vi "NM GlobalTest.vi"() -> ()   [LabVIEW 2010] (continued)
            tunnel: [_ w3958] -> w3939
            tunnel: [_ w3957] -> w3938
            tunnel: [_ w3956] -> w3937
            tunnel: w3936 -> [w3946 _]
            tunnel: [FALSE _] -> w3935
            frame #0 {
              n819 = for {
                N: 5 -> [_]
                tunnel: w3946 -> [w3954]
                n820 = Wait Until Next ms Multiple(millisecond multiple=w3954) -> ()  [unwired: 1 out]
                "Props" <- TRUE
              }
              n821 = case shown="\"DAQmx\"" w3944 {
                frame "ULx", Default {
                }
                frame "DAQmx" {
                  n822 = local write "Burst"("Burst 2") -> ()
                  n823 = local write "Edge"("Edge 2") -> ()
                  n824 = local write "Type"("Type 2") -> ()
                  n825 = local write "SIO"("SIO 2") -> ()
                  n826 = local write "DoWord"("DoWord 2") -> ()
                  n827 = local write "DiWord"("Word 2") -> ()
                }
              }
            }
            frame #1 {
              n828 = case shown="\"Get Properties\", Default" "GetSet" {
                tunnel: w3960 -> [w3970 w5157]
                tunnel: w3962 -> [w3969 w5161]
                tunnel: w3959 -> [w3968 w5160]
                tunnel: w3961 -> [w3967 w5156]
                tunnel: [w3966 w5154] -> w3958
                tunnel: [w3964 w5158] -> w3956
                tunnel: [w3965 w5159] -> w3957
                frame "Get Properties", Default {
                  n829 = stacked-sequence {
                    seq-local: [w3976 _] -> [_ w4127]
                    seq-local: [w3975 _] -> [_ w4126]
                    seq-local: [w3974 _] -> [_ w4125]
                    tunnel: w3970 -> [w3978 _]
                    tunnel: w3969 -> [w3973 w4129]
                    tunnel: w3968 -> [w3972 _]
                    tunnel: w3967 -> [w3977 _]
                    tunnel: [_ w4128] -> w3966
                    tunnel: [_ w4124] -> w3965
                    tunnel: [_ w4123] -> w3964
                    frame #0 {
                      n830 = for {
                        N: 3 -> [_]
                        tunnel: w3973 -> [w3989]
                        shift-right: [w3983] -> w3976
                        shift-left: w3972 -> [w3980]
                        shift-right: [w3984] -> w3975
                        shift-left: w3978 -> [w3981]
                        shift-right: [w3985] -> w3974
                        shift-left: w3977 -> [w3994]
                        i -> [w3993]
                        n831 = case shown="2" w3993 {
                          tunnel: [w4019 w4023 w4027] -> w3992
                          frame 0, Default {
                            n832 = Select(t=1, s="Chans", f=0) -> (s? t:f=w4019:i32)
                          }
                          frame 1 {
                            n833 = Select(t=2, s="Done 2", f=0) -> (s? t:f=w4023:i32)
                          }
                          frame 2 {
                            n834 = Select(t=3, s="Err", f=0) -> (s? t:f=w4027:i32)
                          }
                        }
                        n835 = Not A Number/Path/Refnum?(number/path/refnum=w3981) -> (NaN/Path/Refnum?=w3979:bool)
                        n836 = Not A Number/Path/Refnum?(number/path/refnum=w3980) -> ()  [unwired: 1 out]
                        n837 = case shown="2" w3992 {
                          tunnel: w3981 -> [w4032 w4042 w4081 w4100]
                          tunnel: w3994 -> [w4031 w4038 w4080 w4102]
                          tunnel: [w4033 w4041 w4079 w4099] -> w3988
                          tunnel: [w4032 w4040 w4078 w4096] -> w3987
                          tunnel: [w4031 w4044 w4077 w4095] -> w3986
                          tunnel: w3989 -> [_ w4039 w4076 w4098]
                          tunnel: w3980 -> [w4033 w4043 w4075 w4101]
                          tunnel: [_ w4037 _ _] -> w3990
                          tunnel: w3979 -> [_ w4035 _ w4094]
                          frame 0, Default {
                          }
                          frame 1 {
                            n838 = case shown="\"ULx\", Default" w4039 {
                              tunnel: w4042 -> [w4053 w4073]
                              tunnel: [w4052 w4068] -> w4036
                              tunnel: [w4051 w4071] -> w4044
                              tunnel: [w4050 w4073] -> w4040
                              tunnel: [w4049 w4069] -> w4041
                              tunnel: w4043 -> [w4049 w4070]
                              tunnel: w4038 -> [w4048 w4072]
                              tunnel: [w4047 w4067] -> w4037
                              tunnel: w4035 -> [w4046 _]
                              tunnel: [w4045 w4066] -> w4034
                              frame "ULx", Default {
                                n839 = case shown="False" w4046 {
                                tunnel: w4053 -> [w4054 w4063]
                                tunnel: [w4056 u32 0 ("NumberOfChannels")] -> w4052
                                tunnel: [w4057 w4064] -> w4051
                                tunnel: [w4058 w4063] -> w4050
                                tunnel: w4048 -> [w4060 w4064]
                                tunnel: [w4059 TRUE ("Done")] -> w4047
                                tunnel: [w4055 ""] -> w4045
                                frame False {
                                n840 = call "TaskProps.vi"("task in"=w4054, "error in (no error)"=w4060) -> ("task out"=w4058:refnum<k24>, "NumberOfChannels"=w4056:u32, "Done"=w4059:bool, "error out"=w4057:errorcluster, "DeviceName"=w4055:string)  [unwired: 1 in]
                                }
                                frame True {
                                }
                                }
                              }
                              frame "DAQmx" {
                                n841 = property class="DAQmx Task"(reference=w4070, error in=w4072) -> (reference out=w4069:refnum<k21>, error out=w4071:errorcluster, "NumChans"=w4068:u32, "Done"=w4067:bool, "Name"=w4066:refnum<k21>)
                              }
                            }
                            "Done" <- w4037
                            "NumChans" <- w4036
                            "DevName" <- w4034
                          }
                          frame 2 {
                            n842 = case shown="\"ULx\", Default" w4076 {
                              tunnel: w4081 -> [w4082 w4093]
                              tunnel: [w4085 w4091] -> w4077
                              tunnel: [w4086 w4093] -> w4078
                              tunnel: [w4087 w4092] -> w4079
                              tunnel: w4075 -> [w4087 w4089]
                              tunnel: w4080 -> [w4083 w4088]
                              tunnel: [w4084 w4090] -> w4074
                              frame "ULx", Default {
                                n843 = call <vilib>:"ULx Is Task Done.vi"("task in"=w4082, "error in"=w4083) -> ("task out"=w4086:refnum<k24>, "task done?"=w4084:bool, "error out"=w4085:errorcluster)  [unwired: 11 in]
                              }
                              frame "DAQmx" {
                                n844 = call <vilib>:"DAQmx Is Task Done.vi"("task/channels in"=w4089, "error in"=w4088) -> ("task out"=w4092:refnum<k21>, "task done?"=w4090:bool, "error out"=w4091:errorcluster)  [unwired: 11 in]
                              }
                            }
                            "IT Done" <- w4074
                          }
                          frame 3 {
                            n845 = case shown="\"ULx\", Default" w4098 {
                              tunnel: w4100 -> [w4110 w4122]
                              tunnel: [w4105 w4120] -> w4095
                              tunnel: [w4104 w4122] -> w4096
                              tunnel: [w4109 w4121] -> w4099
                              tunnel: w4101 -> [w4109 w4121]
                              tunnel: w4102 -> [w4108 w4120]
                              tunnel: [w4107 w4119] -> w4097
                              tunnel: w4094 -> [w4103 _]
                              frame "ULx", Default {
                                n846 = case shown="False" w4103 {
                                tunnel: w4110 -> [w4115 w4118]
                                tunnel: w4108 -> [w4114 w4117]
                                tunnel: [w4113 0 ("ErrorCode")] -> w4107
                                tunnel: [w4112 w4117] -> w4106
                                tunnel: [w4111 w4118] -> w4104
                                frame False {
                                n847 = property class="IOTask"(reference=w4115, error in=w4114) -> (reference out=w4111:refnum<k24>, error out=w4112:errorcluster, "ErrorCode"=w4113:i32)
                                }
                                frame True {
                                }
                                }
                                n848 = call <vilib>:"ULx Get Error Info.vi"("error in"=w4106, "ErrorCode"=w4107, "task in"=w4104) -> ("error out"=w4105:errorcluster)  [unwired: 8 in]
                              }
                              frame "DAQmx" {
                                n849 = Unbundle By Name(w4120) -> ("code"=w4119:i32)
                              }
                            }
                            "ErrorCode" <- w4097
                          }
                        }
                        n850 = And(x=w3990, y="Restart\nWhen\nDone") -> (x .and. y?=w3991:bool)
                        n851 = case shown="True" w3991 {
                          tunnel: w3989 -> [_ w4004]
                          tunnel: w3988 -> [w3997 w4001]
                          tunnel: w3987 -> [w3996 w4000]
                          tunnel: w3986 -> [w3995 w4003]
                          tunnel: [w3995 w4002] -> w3985
                          tunnel: [w3997 w3999] -> w3983
                          tunnel: [w3996 w3998] -> w3984
                          frame False {
                          }
                          frame True {
                            n852 = case shown="\"ULx\", Default" w4004 {
                              tunnel: w4003 -> [w4007 w4015]
                              tunnel: [w4011 w4018] -> w4002
                              tunnel: w4001 -> [w4010 w4013]
                              tunnel: [w4010 w4017] -> w3999
                              tunnel: w4000 -> [w4008 w4016]
                              tunnel: [w4009 w4016] -> w3998
                              frame "ULx", Default {
                                n853 = call <vilib>:"ULx Stop Task.vi"("error in"=w4007, "task in"=w4008) -> ("error out"=w4005:errorcluster, "task out"=w4006:refnum<k24>)  [unwired: 8 in]
                                n854 = call <vilib>:"ULx Start Task.vi"("task in"=w4006, "error in"=w4005) -> ("task out"=w4009:refnum<k24>, "error out"=w4011:errorcluster)  [unwired: 12 in]
                              }
                              frame "DAQmx" {
                                n855 = call <vilib>:"DAQmx Stop Task.vi"("task/channels in"=w4013, "error in"=w4015) -> ("task out"=w4012:refnum<k21>, "error out"=w4014:errorcluster)  [unwired: 12 in]
                                n856 = call <vilib>:"DAQmx Start Task.vi"("task/channels in"=w4012, "error in"=w4014) -> ("task out"=w4017:refnum<k21>, "error out"=w4018:errorcluster)  [unwired: 12 in]
                              }
                            }
                          }
                        }
                      }
                    }
                    frame #1 {
                      n857 = case shown="\"Read\", Default" "GetLev" {
                        tunnel: w4126 -> [w4132 w4367 w4557 w4752 w4904 w4953 w5108]
                        tunnel: w4129 -> [w4138 w4369 w4552 w4747 w4902 w4948 w5103]
                        tunnel: w4127 -> [w4133 w4366 w4558 w4753 w4905 w4952 w5109]
                        tunnel: w4125 -> [w4131 w4368 w4556 w4751 w4903 w4954 w5107]
                        tunnel: [w4137 w4363 w4553 w4748 w4899 w4950 w5104] -> w4128
                        tunnel: [w4135 w4365 w4555 w4750 w4901 w4951 w5106] -> w4124
                        tunnel: [w4134 w4364 w4554 w4749 w4900 w4949 w5105] -> w4123
                        frame "Read", Default {
                          n858 = for {
                            N: 8 -> [_]
                            tunnel: w4138 -> [w4147]
                            shift-right: [w4143] -> w4135
                            shift-left: w4133 -> [w4141]
                            shift-right: [w4142] -> w4134
                            shift-left: w4132 -> [w4140]
                            shift-right: [w4146] -> w4137
                            shift-left: w4131 -> [w4139]
                            i -> [w4145]
                            n859 = case shown="0, Default" w4145 {
                              tunnel: [w4148 w4155 w4157 w4160 w4164 w4168 w4173 w4176] -> w4144
                              frame 0, Default {
                                n860 = Select(t=1, s="AutoS", f=0) -> (s? t:f=w4148:i32)
                              }
                              frame 1 {
                                n861 = Select(t=2, s="Avail", f=0) -> (s? t:f=w4155:i32)
                              }
                              frame 2 {
                                n862 = Select(t=3, s="Position", f=0) -> (s? t:f=w4157:i32)
                              }
                              frame 3 {
                                n863 = Select(t=4, s="OWrite", f=0) -> (s? t:f=w4160:i32)
                              }
                              frame 4 {
                                n864 = Select(t=5, s="ReadAll", f=0) -> (s? t:f=w4164:i32)
                              }
                              frame 5 {
                                n865 = Select(t=6, s="Total", f=0) -> (s? t:f=w4168:i32)
                              }
                              frame 6 {
                                n866 = Select(t=7, s="Raw", f=0) -> (s? t:f=w4173:i32)
                              }
                              frame 7 {
                                n867 = Select(t=8, s="Bools", f=0) -> (s? t:f=w4176:i32)
                              }
                            }
                            n868 = case shown="2" w4144 {
                              tunnel: w4147 -> [w4183 w4200 w4219 w4249 w4266 w4289 w4309 w4329 w4346]
                              tunnel: w4140 -> [w4185 w4199 w4222 w4251 w4271 w4291 w4311 w4331 w4348]
                              tunnel: w4139 -> [w4184 w4198 w4221 w4250 w4270 w4290 w4310 w4330 w4347]
                              tunnel: [w4182 w4197 w4218 w4248 w4267 w4286 w4306 w4326 w4343] -> w4146
                              tunnel: w4141 -> [w4186 w4195 w4223 w4252 w4272 w4292 w4312 w4332 w4349]
                              tunnel: [w4181 w4194 w4217 w4247 w4269 w4288 w4308 w4328 w4345] -> w4143
                              tunnel: [w4180 w4193 w4216 w4246 w4268 w4287 w4307 w4327 w4344] -> w4142
                              frame 0, Default {
                                n869 = case shown="\"ULx\", Default" w4183 {
                                tunnel: w4185 -> [w4188 w4192]
                                tunnel: [w4187 w4190] -> w4182
                                tunnel: [w4188 w4192] -> w4180
                                tunnel: [w4189 w4191] -> w4181
                                tunnel: w4186 -> [w4189 w4191]
                                tunnel: w4184 -> [w4187 w4190]
                                frame "ULx", Default {
                                }
                                frame "DAQmx" {
                                }
                                }
                              }
                              frame 1 {
                                n870 = case shown="\"ULx\", Default" w4200 {
                                tunnel: w4199 -> [w4204 w4212]
                                tunnel: [w4201 w4210] -> w4197
                                tunnel: [w4202 w4212] -> w4193
                                tunnel: [w4206 w4208] -> w4194
                                tunnel: w4195 -> [w4206 w4209]
                                tunnel: w4198 -> [w4203 w4211]
                                tunnel: [w4205 w4207] -> w4196
                                frame "ULx", Default {
                                n871 = call "ReadAutoStart.vi"("error in (no error)"=w4203, "task in"=w4204) -> ("error out"=w4201:errorcluster, "AutoStart"=w4205:bool, "task out"=w4202:refnum<k24>)  [unwired: 1 in]
                                }
                                frame "DAQmx" {
                                n872 = property class="DAQmx Read"(reference=w4209, error in=w4211) -> (reference out=w4208:refnum<k21>, error out=w4210:errorcluster, "AutoStart"=w4207:bool)
                                }
                                }
                                "AutoStart" <- w4196
                              }
                              frame 2 {
                                n873 = case shown="\"ULx\", Default" w4219 {
                                tunnel: w4222 -> [w4233 w4244]
                                tunnel: [w4231 w4242] -> w4218
                                tunnel: [w4232 w4244] -> w4216
                                tunnel: [w4234 w4240] -> w4217
                                tunnel: w4223 -> [w4234 w4241]
                                tunnel: w4221 -> [w4230 w4243]
                                tunnel: [w4229 w4239] -> w4220
                                tunnel: [w4228 w4238] -> w4213
                                tunnel: "x" -> [w4227 w4236]
                                tunnel: "Read when Available Samples is greater than this" -> [w4225 w4237]
                                frame "ULx", Default {
                                n874 = call "AvailableSamps.vi"("error in (no error)"=w4230, "task in"=w4233) -> ("error out"=w4231:errorcluster, "AvailableSamples"=w4229:u32, "task out"=w4232:refnum<k24>)  [unwired: 1 in]
                                n875 = Greater?(x=w4229, y=w4225) -> (0:w4226:bool)
                                n876 = And(x=w4226, y=w4227) -> (x .and. y?=w4228:bool)
                                }
                                frame "DAQmx" {
                                n877 = property class="DAQmx Read"(reference=w4241, error in=w4243) -> (reference out=w4240:refnum<k21>, error out=w4242:errorcluster, "AvailSampPerChan"=w4239:u32)
                                n878 = Greater?(x=w4239, y=w4237) -> (0:w4235:bool)
                                n879 = And(x=w4235, y=w4236) -> (x .and. y?=w4238:bool)
                                }
                                }
                                "Available Samples" <- w4220
                                n880 = case shown="True" w4213 {
                                frame False {
                                }
                                frame True {
                                n881 = local write "Read"(TRUE ("Read")) -> ()
                                }
                                }
                              }
                              frame 3 {
                                n882 = case shown="\"ULx\", Default" w4249 {
                                tunnel: w4251 -> [w4254 w4264]
                                tunnel: [w4255 w4262] -> w4248
                                tunnel: [w4253 w4264] -> w4246
                                tunnel: [w4258 w4260] -> w4247
                                tunnel: w4252 -> [w4258 w4261]
                                tunnel: w4250 -> [w4256 w4263]
                                tunnel: [w4257 w4259] -> w4245
                                frame "ULx", Default {
                                n883 = call "CurrentReadPosition.vi"("error in (no error)"=w4256, "task in"=w4254) -> ("error out"=w4255:errorcluster, "CurrReadPosition"=w4257:u32, "task out"=w4253:refnum<k24>)  [unwired: 1 in]
                                }
                                frame "DAQmx" {
                                n884 = property class="DAQmx Read"(reference=w4261, error in=w4263) -> (reference out=w4260:refnum<k21>, error out=w4262:errorcluster, "CurrReadPos"=w4259:dbl)
                                }
                                }
                                "CurrReadPos" <- w4245
                              }
                              frame 4 {
                                n885 = case shown="\"ULx\", Default" w4266 {
                                tunnel: w4271 -> [w4275 w4284]
                                tunnel: [w4274 w4282] -> w4267
                                tunnel: [w4275 w4284] -> w4268
                                tunnel: [w4276 w4280] -> w4269
                                tunnel: w4272 -> [w4276 w4281]
                                tunnel: w4270 -> [w4274 w4283]
                                tunnel: [TRUE w4277] -> w4265
                                frame "ULx", Default {
                                }
                                frame "DAQmx" {
                                w4279 = 10252 items=["Overwrite Unread Samples"=10252, "Do Not Overwrite Unread Samples"=10159] ("OverWrite")
                                n886 = property class="DAQmx Read"(reference=w4281, error in=w4283) -> (reference out=w4280:refnum<k21>, error out=w4282:errorcluster, "OverWrite"=w4278:i32)
                                n887 = Equal?(x=w4278, y=w4279) -> (x = y?=w4277:bool)
                                }
                                }
                                "OverWrite" <- w4265
                              }
                              frame 5 {
                                n888 = case shown="\"ULx\", Default" w4289 {
                                tunnel: w4291 -> [w4294 w4304]
                                tunnel: [w4295 w4302] -> w4286
                                tunnel: [w4293 w4304] -> w4287
                                tunnel: [w4298 w4300] -> w4288
                                tunnel: w4292 -> [w4298 w4301]
                                tunnel: w4290 -> [w4296 w4303]
                                tunnel: [w4297 w4299] -> w4285
                                frame "ULx", Default {
                                n889 = call "ReadAllData.vi"("error in (no error)"=w4296, "task in"=w4294) -> ("error out"=w4295:errorcluster, "ReadAll"=w4297:bool, "task out"=w4293:refnum<k24>)  [unwired: 1 in]
                                }
                                frame "DAQmx" {
                                n890 = property class="DAQmx Read"(reference=w4301, error in=w4303) -> (reference out=w4300:refnum<k21>, error out=w4302:errorcluster, "ReadAllAvailSamp"=w4299:bool)
                                }
                                }
                                "ReadAllAvailSamp" <- w4285
                              }
                              frame 6 {
                                n891 = case shown="\"ULx\", Default" w4309 {
                                tunnel: w4311 -> [w4315 w4324]
                                tunnel: [w4313 w4322] -> w4306
                                tunnel: [w4314 w4324] -> w4307
                                tunnel: [w4318 w4320] -> w4308
                                tunnel: w4312 -> [w4318 w4321]
                                tunnel: w4310 -> [w4316 w4323]
                                tunnel: [w4317 w4319] -> w4305
                                frame "ULx", Default {
                                n892 = call "TotalAcquired.vi"("error in (no error)"=w4316, "task in"=w4315) -> ("error out"=w4313:errorcluster, "TotalAcquired"=w4317:u32, "task out"=w4314:refnum<k24>)  [unwired: 1 in]
                                }
                                frame "DAQmx" {
                                n893 = property class="DAQmx Read"(reference=w4321, error in=w4323) -> (reference out=w4320:refnum<k21>, error out=w4322:errorcluster, "TotalSampPerChanAcquired"=w4319:dbl)
                                }
                                }
                                "TotalPerAcquired" <- w4305
                              }
                              frame 7 {
                                n894 = case shown="\"ULx\", Default" w4329 {
                                tunnel: w4331 -> [w4335 w4341]
                                tunnel: [w4333 w4340] -> w4326
                                tunnel: [w4334 w4341] -> w4327
                                tunnel: [w4338 w4339] -> w4328
                                tunnel: w4332 -> [w4338 w4339]
                                tunnel: w4330 -> [w4336 w4340]
                                tunnel: [w4337 _] -> w4325
                                frame "ULx", Default {
                                n895 = call "ReadRawData.vi"("error in (no error)"=w4336, "task in"=w4335) -> ("error out"=w4333:errorcluster, "ReadRaw"=w4337:bool, "task out"=w4334:refnum<k24>)  [unwired: 1 in]
                                }
                                frame "DAQmx" {
                                }
                                }
                                "RawData" <- w4325
                              }
                              frame 8 {
                                n896 = case shown="\"ULx\", Default" w4346 {
                                tunnel: w4348 -> [w4353 w4361]
                                tunnel: [w4350 w4359] -> w4343
                                tunnel: [w4352 w4361] -> w4344
                                tunnel: [w4355 w4358] -> w4345
                                tunnel: w4349 -> [w4355 w4357]
                                tunnel: w4347 -> [w4351 w4360]
                                tunnel: [w4354 w4356] -> w4342
                                frame "ULx", Default {
                                n897 = call "NumberOfBools.vi"("error in (no error)"=w4351, "task in"=w4353) -> ("error out"=w4350:errorcluster, "NumberOfBools"=w4354:u32, "task out"=w4352:refnum<k24>)  [unwired: 1 in]
                                }
                                frame "DAQmx" {
                                n898 = property class="DAQmx Channel"(reference=w4357, error in=w4360) -> (reference out=w4358:refnum<k21>, error out=w4359:errorcluster, "DI.NumLines"=w4356:u32)
                                }
                                }
                                "NumberOfBoolsPer" <- w4342
                              }
                            }
                          }
                        }
                        frame "Write" {
                          n899 = for {
                            N: 7 -> [_]
                            tunnel: w4369 -> [w4378]
                            shift-right: [w4374] -> w4365
                            shift-left: w4366 -> [w4375]
                            shift-right: [w4373] -> w4364
                            shift-left: w4367 -> [w4376]
                            shift-right: [w4372] -> w4363
                            shift-left: w4368 -> [w4377]
                            i -> [w4371]
                            n900 = case shown="6" w4371 {
                              tunnel: [w4379 w4383 w4387 w4391 w4395 w4399 w4403] -> w4370
                              frame 0, Default {
                                n901 = Select(t=1, s="WrtPos", f=0) -> (s? t:f=w4379:i32)
                              }
                              frame 1 {
                                n902 = Select(t=2, s="Reg 2", f=0) -> (s? t:f=w4383:i32)
                              }
                              frame 2 {
                                n903 = Select(t=3, s="Gen", f=0) -> (s? t:f=w4387:i32)
                              }
                              frame 3 {
                                n904 = Select(t=4, s="Space", f=0) -> (s? t:f=w4391:i32)
                              }
                              frame 4 {
                                n905 = Select(t=5, s="Bools 2", f=0) -> (s? t:f=w4395:i32)
                              }
                              frame 5 {
                                n906 = Select(t=6, s="RelTo", f=0) -> (s? t:f=w4399:i32)
                              }
                              frame 6 {
                                n907 = Select(t=7, s="Offset", f=0) -> (s? t:f=w4403:i32)
                              }
                            }
                            n908 = case shown="4" w4370 {
                              tunnel: w4378 -> [_ w4417 w4434 w4456 w4477 w4507 w4523 w4539]
                              tunnel: w4377 -> [w4407 w4416 w4435 w4457 w4478 w4506 w4524 w4540]
                              tunnel: w4376 -> [w4408 w4415 w4436 w4458 w4479 w4505 w4525 w4541]
                              tunnel: w4375 -> [w4409 w4414 w4437 w4459 w4480 w4504 w4526 w4542]
                              tunnel: [w4409 w4413 w4433 w4455 w4476 w4503 w4522 w4538] -> w4374
                              tunnel: [w4408 w4412 w4432 w4454 w4475 w4502 w4521 w4537] -> w4373
                              tunnel: [w4407 w4411 w4431 w4453 w4474 w4501 w4520 w4536] -> w4372
                              frame 0, Default {
                              }
                              frame 1 {
                                n909 = case shown="\"ULx\", Default" w4417 {
                                tunnel: w4415 -> [w4419 w4429]
                                tunnel: [w4420 w4427] -> w4411
                                tunnel: [w4418 w4429] -> w4412
                                tunnel: [w4423 w4425] -> w4413
                                tunnel: w4414 -> [w4423 w4426]
                                tunnel: w4416 -> [w4421 w4428]
                                tunnel: [w4422 w4424] -> w4410
                                frame "ULx", Default {
                                n910 = call "CurrWritePos.vi"("error in (no error)"=w4421, "task in"=w4419) -> ("error out"=w4420:errorcluster, "CurrWritePos"=w4422:u32, "task out"=w4418:refnum<k24>)  [unwired: 1 in]
                                }
                                frame "DAQmx" {
                                n911 = property class="DAQmx Write"(reference=w4426, error in=w4428) -> (reference out=w4425:refnum<k21>, error out=w4427:errorcluster, "CurrWritePos"=w4424:dbl)
                                }
                                }
                                "CurrentWritePosition" <- w4410
                              }
                              frame 2 {
                                n912 = case shown="\"ULx\", Default" w4434 {
                                tunnel: w4436 -> [w4440 w4451]
                                tunnel: [w4438 w4449] -> w4431
                                tunnel: [w4439 w4451] -> w4432
                                tunnel: [w4443 w4447] -> w4433
                                tunnel: w4437 -> [w4443 w4448]
                                tunnel: w4435 -> [w4441 w4450]
                                tunnel: [w4442 w4444] -> w4430
                                frame "ULx", Default {
                                n913 = call "WriteRegen.vi"("error in (no error)"=w4441, "task in"=w4440) -> ("error out"=w4438:errorcluster, "Regenerate"=w4442:bool, "task out"=w4439:refnum<k24>)  [unwired: 1 in]
                                }
                                frame "DAQmx" {
                                w4446 = 10097 items=["Allow Regeneration"=10097, "Do Not Allow Regeneration"=10158] ("RegenMode")
                                n914 = property class="DAQmx Write"(reference=w4448, error in=w4450) -> (reference out=w4447:refnum<k21>, error out=w4449:errorcluster, "RegenMode"=w4445:i32)
                                n915 = Equal?(x=w4445, y=w4446) -> (x = y?=w4444:bool)
                                }
                                }
                                "Regenerate" <- w4430
                              }
                              frame 3 {
                                n916 = case shown="\"ULx\", Default" w4456 {
                                tunnel: w4458 -> [w4461 w4471]
                                tunnel: [w4462 w4469] -> w4453
                                tunnel: [w4460 w4471] -> w4454
                                tunnel: [w4465 w4467] -> w4455
                                tunnel: w4459 -> [w4465 w4468]
                                tunnel: w4457 -> [w4463 w4470]
                                tunnel: [w4464 w4466] -> w4452
                                frame "ULx", Default {
                                n917 = call "SamplesGenerated.vi"("error in (no error)"=w4463, "task in"=w4461) -> ("error out"=w4462:errorcluster, "SamplesGenerated"=w4464:u32, "task out"=w4460:refnum<k24>)  [unwired: 1 in]
                                }
                                frame "DAQmx" {
                                n918 = property class="DAQmx Write"(reference=w4468, error in=w4470) -> (reference out=w4467:refnum<k21>, error out=w4469:errorcluster, "TotalSampPerChanGenerated"=w4466:dbl)
                                }
                                }
                                "Generated" <- w4452
                              }
                              frame 4 {
                                n919 = case shown="\"ULx\", Default" w4477 {
                                tunnel: w4479 -> [w4488 w4499]
                                tunnel: [w4490 w4497] -> w4474
                                tunnel: [w4489 w4499] -> w4475
                                tunnel: [w4491 w4495] -> w4476
                                tunnel: w4480 -> [w4491 w4496]
                                tunnel: w4478 -> [w4487 w4498]
                                tunnel: [w4482 w4494] -> w4473
                                tunnel: [w4481 w4492] -> w4472
                                frame "ULx", Default {
                                n920 = property class="IOTask"(reference=w4488, error in=w4487) -> (reference out=w4486:refnum<k24>, error out=w4485:errorcluster, "Write.SpaceAvailable"=w4481:u32)
                                n921 = call "SpaceAvailable.vi"("error in (no error)"=w4485, "task in"=w4486) -> ("error out"=w4490:errorcluster, "SpaceAvailable"=w4483:u32, "task out"=w4489:refnum<k24>)  [unwired: 1 in]
                                "CWP - Generated" <- w4483
                                n922 = Less?(x=w4483, y="Write when \"CWP - Generated\" < this number.") -> (x < y?=w4482:bool)
                                }
                                frame "DAQmx" {
                                n923 = property class="DAQmx Write"(reference=w4496, error in=w4498) -> (reference out=w4495:refnum<k21>, error out=w4497:errorcluster, "SpaceAvail"=w4492:u32)
                                n924 = Greater?(x=w4492, y="Write when SA > this.") -> (0:w4494:bool)
                                }
                                }
                                "SpaceAvailable" <- w4472
                                n925 = local write "Write"(w4473) -> ()
                              }
                              frame 5 {
                                n926 = case shown="\"ULx\", Default" w4507 {
                                tunnel: w4505 -> [w4510 w4519]
                                tunnel: [w4508 w4516] -> w4501
                                tunnel: [w4509 w4519] -> w4502
                                tunnel: [w4513 w4515] -> w4503
                                tunnel: w4504 -> [w4513 w4517]
                                tunnel: w4506 -> [w4511 w4518]
                                tunnel: [w4512 w4514] -> w4500
                                frame "ULx", Default {
                                n927 = call "NumberOfBoolsWr.vi"("error in (no error)"=w4511, "task in"=w4510) -> ("error out"=w4508:errorcluster, "NumBoolsWr"=w4512:u32, "task out"=w4509:refnum<k24>)  [unwired: 1 in]
                                }
                                frame "DAQmx" {
                                n928 = property class="DAQmx Write"(reference=w4517, error in=w4518) -> (reference out=w4515:refnum<k21>, error out=w4516:errorcluster, "DO.NumBooleansPerChan"=w4514:u32)
                                }
                                }
                                "BooleansPer" <- w4500
                              }
                              frame 6 {
                                n929 = case shown="\"ULx\", Default" w4523 {
                                tunnel: w4525 -> [w4527 w4535]
                                tunnel: [w4528 w4533] -> w4520
                                tunnel: [w4527 w4535] -> w4521
                                tunnel: [w4529 w4531] -> w4522
                                tunnel: w4526 -> [w4529 w4532]
                                tunnel: w4524 -> [w4528 w4534]
                                frame "ULx", Default {
                                }
                                frame "DAQmx" {
                                n930 = property class="DAQmx Write"(reference=w4532, error in=w4534) -> (reference out=w4531:refnum<k21>, error out=w4533:errorcluster, "RelativeTo"=→"RelativeTo":i32)
                                }
                                }
                              }
                              frame 7 {
                                n931 = case shown="\"ULx\", Default" w4539 {
                                tunnel: w4541 -> [w4543 w4551]
                                tunnel: [w4544 w4549] -> w4536
                                tunnel: [w4543 w4551] -> w4537
                                tunnel: [w4545 w4547] -> w4538
                                tunnel: w4542 -> [w4545 w4548]
                                tunnel: w4540 -> [w4544 w4550]
                                frame "ULx", Default {
                                }
                                frame "DAQmx" {
                                n932 = property class="DAQmx Write"(reference=w4548, error in=w4550) -> (reference out=w4547:refnum<k21>, error out=w4549:errorcluster, "Offset"=→"Offset":i32)
                                }
                                }
                              }
                            }
                          }
                        }
                        frame "Trigger" {
                          n933 = stacked-sequence {
                            seq-local: [w4561 _] -> [_ w4578]
                            seq-local: [w4560 _] -> [_ w4577]
                            seq-local: [w4559 _] -> [_ w4576]
                            tunnel: w4558 -> [w4562 _]
                            tunnel: w4557 -> [w4563 _]
                            tunnel: w4556 -> [w4564 _]
                            tunnel: [_ w4582] -> w4555
                            tunnel: [_ w4581] -> w4554
                            tunnel: [_ w4580] -> w4553
                            tunnel: w4552 -> [w4565 w4579]
                            frame #0 {
                              n934 = case shown="\"ULx\", Default" w4565 {
                                tunnel: w4563 -> [w4570 w4574]
                                tunnel: [w4567 w4572] -> w4559
                                tunnel: [w4566 w4574] -> w4560
                                tunnel: [w4571 w4573] -> w4561
                                tunnel: w4562 -> [w4571 w4573]
                                tunnel: w4564 -> [w4568 w4572]
                                frame "ULx", Default {
                                n935 = call "TrigMode.vi"("error in (no error)"=w4568, "task in"=w4570) -> ("error out"=w4567:errorcluster, "TrigMode"=→"Mode":i32, "task out"=w4566:refnum<k24>)  [unwired: 1 in]
                                }
                                frame "DAQmx" {
                                }
                              }
                            }
                            frame #1 {
                              n936 = case shown="\"Basic\", Default" "GtULxTrgP" {
                                tunnel: [w4590 w4674 w4700 w4728] -> w4582
                                tunnel: [w4589 w4673 w4699 w4725] -> w4581
                                tunnel: [w4588 w4672 w4698 w4723] -> w4580
                                tunnel: w4579 -> [w4587 w4675 w4697 w4727]
                                tunnel: w4578 -> [w4585 w4678 w4703 w4729]
                                tunnel: w4577 -> [w4584 w4677 w4702 w4726]
                                tunnel: w4576 -> [w4583 w4676 w4701 w4724]
                                frame "Basic", Default {
                                n937 = for {
                                N: 3 -> [_]
                                shift-right: [w4596] -> w4590
                                shift-left: w4585 -> [w4599]
                                shift-right: [w4595] -> w4589
                                shift-left: w4584 -> [w4598]
                                shift-right: [w4594] -> w4588
                                shift-left: w4583 -> [w4597]
                                tunnel: w4587 -> [w4593]
                                i -> [w4592]
                                n938 = case shown="2" w4592 {
                                tunnel: [w4660 w4664 w4668] -> w4591
                                frame 0, Default {
                                n939 = Select(t=1, s="Type", f=0) -> (s? t:f=w4660:i32)
                                }
                                frame 1 {
                                n940 = Select(t=2, s="Edge", f=0) -> (s? t:f=w4664:i32)
                                }
                                frame 2 {
                                n941 = Select(t=3, s="Other", f=0) -> (s? t:f=w4668:i32)
                                }
                                }
                                n942 = case shown="1" w4591 {
                                tunnel: w4599 -> [w4602 w4609 w4625 w4642]
                                tunnel: w4598 -> [w4601 w4608 w4626 w4645]
                                tunnel: w4597 -> [w4600 w4607 w4627 w4646]
                                tunnel: [w4602 w4606 w4624 w4641] -> w4596
                                tunnel: [w4601 w4605 w4623 w4643] -> w4595
                                tunnel: [w4600 w4604 w4622 w4644] -> w4594
                                tunnel: w4593 -> [_ w4603 w4628 w4647]
                                frame 0, Default {
                                }
                                frame 1 {
                                n943 = case shown="\"ULx\", Default" w4603 {
                                tunnel: w4608 -> [w4611 w4621]
                                tunnel: [w4612 w4619] -> w4604
                                tunnel: [w4610 w4621] -> w4605
                                tunnel: [w4615 w4617] -> w4606
                                tunnel: w4609 -> [w4615 w4618]
                                tunnel: w4607 -> [w4613 w4620]
                                frame "ULx", Default {
                                n944 = call "TrigBasicType.vi"("error in (no error)"=w4613, "task in"=w4611) -> ("error out"=w4612:errorcluster, "TrigType"=→"Type":i32, "task out"=w4610:refnum<k24>)  [unwired: 1 in]
                                }
                                frame "DAQmx" {
                                n945 = property class="DAQmx Trigger"(reference=w4618, error in=w4620) -> (reference out=w4617:refnum<k21>, error out=w4619:errorcluster, "Start:Trigger Type"=→"TrigType":i32)
                                }
                                }
                                }
                                frame 2 {
                                n946 = case shown="\"ULx\", Default" w4628 {
                                tunnel: w4626 -> [w4630 w4640]
                                tunnel: [w4631 w4638] -> w4622
                                tunnel: [w4629 w4640] -> w4623
                                tunnel: [w4634 w4636] -> w4624
                                tunnel: w4625 -> [w4634 w4637]
                                tunnel: w4627 -> [w4632 w4639]
                                frame "ULx", Default {
                                n947 = call "TrigBasicEdge.vi"("error in (no error)"=w4632, "task in"=w4630) -> ("error out"=w4631:errorcluster, "TrigEdge"=→"Edge":i32, "task out"=w4629:refnum<k24>)  [unwired: 1 in]
                                }
                                frame "DAQmx" {
                                n948 = property class="DAQmx Trigger"(reference=w4637, error in=w4639) -> (reference out=w4636:refnum<k21>, error out=w4638:errorcluster, "Start.DigEdge.Edge"=→"DigEdge.Edge":i32)
                                }
                                }
                                }
                                frame 3 {
                                n949 = case shown="\"ULx\", Default" w4647 {
                                tunnel: w4646 -> [w4654 w4658]
                                tunnel: w4645 -> [w4653 w4659]
                                tunnel: [w4651 w4658] -> w4644
                                tunnel: [w4652 w4659] -> w4643
                                tunnel: w4642 -> [w4656 w4657]
                                tunnel: [w4656 w4657] -> w4641
                                frame "ULx", Default {
                                n950 = call "TrigBasicProps.vi"("task in"=w4653, "error in (no error)"=w4654) -> ("Slope"=→"Slope":i32, "PretriggerCount"=→"PretriggerCount":i32, "task out"=w4652:refnum<k24>, "DigLevel"=→"DigitalLevel":i32, "AnalogLevel"=→"AnalogLevel":dbl, "error out"=w4651:errorcluster)  [unwired: 1 in]
                                }
                                frame "DAQmx" {
                                }
                                }
                                }
                                }
                                }
                                }
                                frame "Gated" {
                                n951 = case shown="\"ULx\", Default" w4675 {
                                tunnel: w4676 -> [w4692 w4695]
                                tunnel: w4677 -> [w4691 w4696]
                                tunnel: [w4689 w4695] -> w4672
                                tunnel: [w4690 w4696] -> w4673
                                tunnel: w4678 -> [w4693 w4694]
                                tunnel: [w4693 w4694] -> w4674
                                frame "ULx", Default {
                                n952 = call "TrigGatedProps.vi"("task in"=w4691, "error in (no error)"=w4692) -> ("When"=→"When":i32, "Hysteresis"=→"Hysteresis":i32, "Position"=→"Position":i32, "WindowBottom"=→"WindowBottom":dbl, "Type"=→"Type":i32, "WindowTop"=→"WindowTop":dbl, "task out"=w4690:refnum<k24>, "AnalogLevel"=→"AnalogLevel":dbl, "DigitalLevel"=→"DigitalLevel":i32, "HighThreshold"=→"HighThreshold":dbl, "LowThreshold"=→"LowThreshold":dbl, "error out"=w4689:errorcluster)  [unwired: 6 in]
                                }
                                frame "DAQmx" {
                                }
                                }
                                }
                                frame "Start" {
                                n953 = case shown="\"ULx\", Default" w4697 {
                                tunnel: w4701 -> [w4718 w4721]
                                tunnel: w4702 -> [w4717 w4722]
                                tunnel: [w4715 w4721] -> w4698
                                tunnel: [w4716 w4722] -> w4699
                                tunnel: w4703 -> [w4719 w4720]
                                tunnel: [w4719 w4720] -> w4700
                                frame "ULx", Default {
                                n954 = call "CompTrigStartProps.vi"("task in"=w4717, "error in (no error)"=w4718) -> ("AnalogHWTrigSense"=→"AnalogHWSense":i32, "TrigChannelStr"=→"TriggerChannelStr":string, "AnalogSWTrigSense"=→"AnalogSWSense":i32, "TriggerChannel"=→"Channel":i32, "CounterChanTrigSense"=→"CounterChannelSense":i32, "Variance"=→"Variance":dbl, "DigitalPatternTrigSense"=→"DigitalPatternSense":i32, "task out"=w4716:refnum<k24>, "Level"=→"Level":dbl, "Type"=→"Type":i32, "PretriggerCount"=→"PretriggerCount":i32, "ExtTTLTrigSense"=→"ExtTTLSense":i32, "error out"=w4715:errorcluster)  [unwired: 5 in]
                                }
                                frame "DAQmx" {
                                }
                                }
                                }
                                frame "Stop" {
                                n955 = case shown="\"ULx\", Default" w4727 {
                                tunnel: [w4738 w4743] -> w4723
                                tunnel: [w4739 w4744] -> w4725
                                tunnel: w4729 -> [w4742 w4745]
                                tunnel: [w4742 w4745] -> w4728
                                tunnel: w4726 -> [w4740 w4744]
                                tunnel: w4724 -> [w4741 w4743]
                                frame "ULx", Default {
                                n956 = call "CompTrigStopProps.vi"("task in"=w4740, "error in (no error)"=w4741) -> ("TriggerChannelStr"=→"TriggerChannelStr":string, "AnalogSWTriggerSense"=→"AnalogSWSense":i32, "TriggerChannel"=→"Channel":i32, "CounterChannelTriggerSense"=→"CounterChannelSense":i32, "Variance"=→"Variance":dbl, "DigitalPatternTriggerSense"=→"DigitalPatternSense":i32, "task out"=w4739:refnum<k24>, "Level"=→"Level":dbl, "Type"=→"Type":i32, "error IO"=w4738:errorcluster)  [unwired: 8 in]
                                }
                                frame "DAQmx" {
                                }
                                }
                                }
                              }
                            }
                          }
                        }
                        frame "Timing" {
                          n957 = for {
                            N: 6 -> [_]
                            shift-right: [w4759] -> w4750
                            shift-left: w4753 -> [w4762]
                            shift-right: [w4758] -> w4749
                            shift-left: w4752 -> [w4761]
                            shift-right: [w4757] -> w4748
                            shift-left: w4751 -> [w4760]
                            tunnel: w4747 -> [w4756]
                            i -> [w4755]
                            n958 = case shown="4" w4755 {
                              tunnel: [w4874 w4878 w4882 w4886 w4891 w4895] -> w4754
                              frame 0, Default {
                                n959 = Select(t=1, s="Burst", f=0) -> (s? t:f=w4874:i32)
                              }
                              frame 1 {
                                n960 = Select(t=2, s="SIO", f=0) -> (s? t:f=w4878:i32)
                              }
                              frame 2 {
                                n961 = Select(t=3, s="DiWord", f=0) -> (s? t:f=w4882:i32)
                              }
                              frame 3 {
                                n962 = Select(t=4, s="DoWord", f=0) -> (s? t:f=w4886:i32)
                              }
                              frame 4 {
                                n963 = Select(t=5, s="Actual Rate", f=0) -> (s? t:f=w4891:i32)
                              }
                              frame 5 {
                                n964 = Select(t=6, s="UFlow", f=0) -> (s? t:f=w4895:i32)
                              }
                            }
                            n965 = case shown="5" w4754 {
                              tunnel: w4762 -> [w4765 w4772 w4786 w4803 w4825 w4845 w4859]
                              tunnel: w4761 -> [w4764 w4771 w4787 w4804 w4823 w4844 w4861]
                              tunnel: w4760 -> [w4763 w4770 w4788 w4805 w4822 w4843 w4863]
                              tunnel: [w4765 w4769 w4785 w4802 w4824 w4841 w4858] -> w4759
                              tunnel: [w4764 w4768 w4784 w4801 w4821 w4840 w4860] -> w4758
                              tunnel: [w4763 w4767 w4783 w4800 w4820 w4839 w4862] -> w4757
                              tunnel: w4756 -> [_ w4766 w4789 w4806 w4819 w4842 w4864]
                              frame 0, Default {
                              }
                              frame 1 {
                                n966 = case shown="\"ULx\", Default" w4766 {
                                tunnel: w4771 -> [w4774 w4782]
                                tunnel: [w4775 w4780] -> w4767
                                tunnel: [w4774 w4782] -> w4768
                                tunnel: [w4776 w4778] -> w4769
                                tunnel: w4772 -> [w4776 w4779]
                                tunnel: w4770 -> [w4775 w4781]
                                frame "ULx", Default {
                                "BurstIO" <- FALSE ("BurstIO")
                                }
                                frame "DAQmx" {
                                n967 = property class="DAQmx Timing"(reference=w4779, error in=w4781) -> (reference out=w4778:refnum<k21>, error out=w4780:errorcluster, "SampTimingType"=→"SampTimingType":i32)
                                }
                                }
                              }
                              frame 2 {
                                n968 = case shown="\"ULx\", Default" w4789 {
                                tunnel: w4787 -> [w4791 w4799]
                                tunnel: [w4792 w4797] -> w4783
                                tunnel: [w4791 w4799] -> w4784
                                tunnel: [w4793 w4795] -> w4785
                                tunnel: w4786 -> [w4793 w4796]
                                tunnel: w4788 -> [w4792 w4798]
                                frame "ULx", Default {
                                "SingleIO" <- FALSE ("SingleIO")
                                }
                                frame "DAQmx" {
                                n969 = property class="DAQmx Timing"(reference=w4796, error in=w4798) -> (reference out=w4795:refnum<k21>, error out=w4797:errorcluster, "SampQuant.SampMode"=→"SampQuant.SampMode":i32)
                                }
                                }
                              }
                              frame 3 {
                                n970 = case shown="\"ULx\", Default" w4806 {
                                tunnel: w4804 -> [w4808 w4818]
                                tunnel: [w4809 w4816] -> w4800
                                tunnel: [w4807 w4818] -> w4801
                                tunnel: [w4812 w4814] -> w4802
                                tunnel: w4803 -> [w4812 w4815]
                                tunnel: w4805 -> [w4810 w4817]
                                frame "ULx", Default {
                                n971 = call "DIWordXfer.vi"("error in (no error)"=w4810, "task in"=w4808) -> ("error out"=w4809:errorcluster, "DIWord"=→"DI.WordTransfer":bool, "task out"=w4807:refnum<k24>)  [unwired: 1 in]
                                }
                                frame "DAQmx" {
                                n972 = property class="DAQmx Timing"(reference=w4815, error in=w4817) -> (reference out=w4814:refnum<k21>, error out=w4816:errorcluster, "SampQuant.SampPerChan"=→"SampQuant.SampPerChan":dbl)
                                }
                                }
                              }
                              frame 4 {
                                n973 = case shown="\"ULx\", Default" w4819 {
                                tunnel: w4823 -> [w4827 w4837]
                                tunnel: [w4828 w4835] -> w4820
                                tunnel: [w4826 w4837] -> w4821
                                tunnel: [w4831 w4833] -> w4824
                                tunnel: w4825 -> [w4831 w4834]
                                tunnel: w4822 -> [w4829 w4836]
                                frame "ULx", Default {
                                n974 = call "DOWordXfer.vi"("error in (no error)"=w4829, "task in"=w4827) -> ("error out"=w4828:errorcluster, "DOWord"=→"DO.WordTransfer":bool, "task out"=w4826:refnum<k24>)  [unwired: 1 in]
                                }
                                frame "DAQmx" {
                                n975 = property class="DAQmx Timing"(reference=w4834, error in=w4836) -> (reference out=w4833:refnum<k21>, error out=w4835:errorcluster, "SampClk.Src"=→"SampClk.Src":tag)
                                }
                                }
                              }
                              frame 5 {
                                n976 = case shown="\"DAQmx\"" w4842 {
                                tunnel: w4844 -> [w4850 w4857]
                                tunnel: [w4848 w4854] -> w4839
                                tunnel: [w4847 w4857] -> w4840
                                tunnel: [w4851 w4852] -> w4841
                                tunnel: w4845 -> [w4851 w4853]
                                tunnel: w4843 -> [w4849 w4855]
                                tunnel: [w4846 w4856] -> w4838
                                frame "ULx", Default {
                                n977 = call "TimingRate.vi"("error in (no error)"=w4849, "task in"=w4850) -> ("error out"=w4848:errorcluster, "ActualRate"=w4846:sgl, "task out"=w4847:refnum<k24>)  [unwired: 1 in]
                                }
                                frame "DAQmx" {
                                n978 = property class="DAQmx Timing"(reference=w4853, error in=w4855) -> (reference out=w4852:refnum<k21>, error out=w4854:errorcluster, "SampClk.Rate"=w4856:dbl)
